vi "Main-National.vi"() -> ()   [LabVIEW 2019]
uses:
  ctl/main data-national.ctl
  ctl/position set.ctl
  ctl/act seq name.ctl
  FPGA_subVIs/low level/DIO/DIO enum.ctl
  ctl/servo act.ctl
  ctl/align type.ctl
  ctl/path name.ctl
  ctl/height.ctl
  subVI/move/position cluster.ctl
  FPGA_subVIs/low level/DIO/DIO.lvclass
  FPGA_subVIs/my FPGA lib.lvlib
panel:
  out "main-national data":T1={"board vision"=[["green", "", "", ""], ["black", "", "", ""], ["", "", "", "yellow"], ["blue", "", "", ""], ["red", "", "", ""]], "recycle room"=[], "box array"=[], "catch array"=[], "put room"="", "catch count"=0.0, "position set"={"vision board"=0.0, "catch box"=0.0, "R1 position"=0.0, "R5 position"=0.0}, "reg data"=[], "S gyro"=0.0}
  out "error out":errorcluster
  in  "error in (no error)":errorcluster
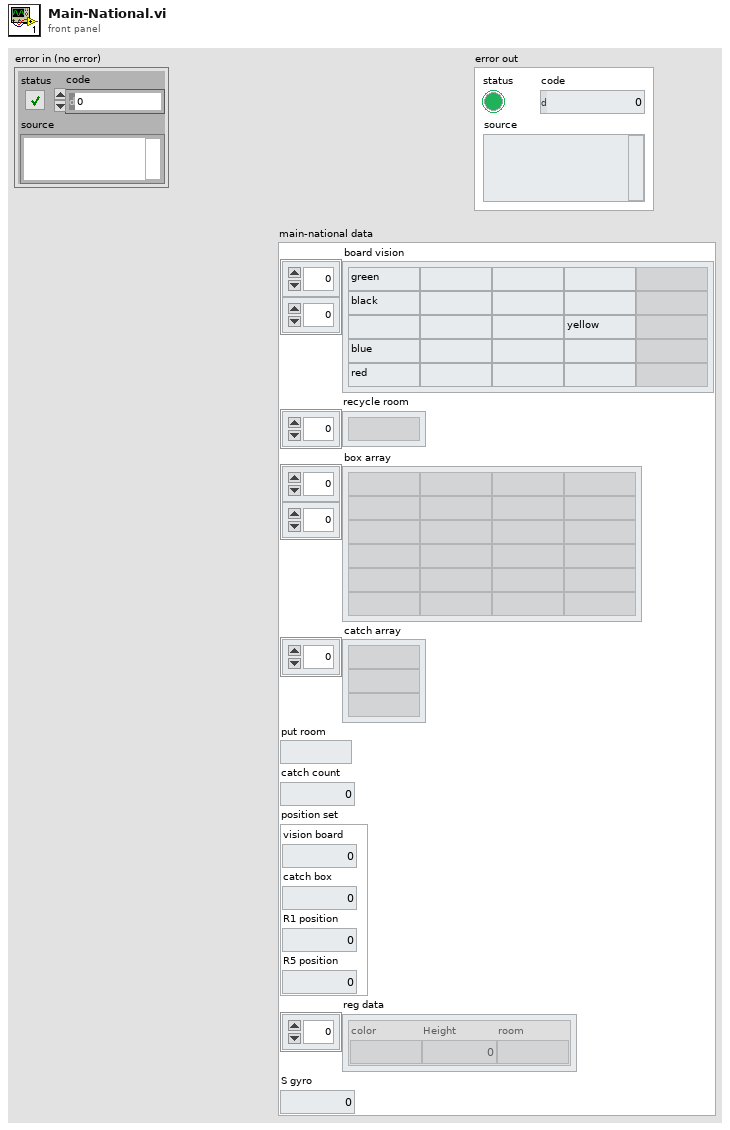
[diagram p1: front panel]
types:
  T1 = typedef "main data-national.ctl" = cluster{"board vision":string[][], "recycle room":string[], "box array":string[][], "catch array":string[], "put room":string, "catch count":dbl, "position set":T2, "reg data":cluster{"color":string, "Height":i32, "room":string}[], "S gyro":dbl}
  T2 = typedef "position set.ctl" = cluster{"vision board":dbl, "catch box":dbl, "R1 position":dbl, "R5 position":dbl}
  T3 = typedef "act seq name.ctl" = enum16{"init", "goto vision board", "go room for get recycle", "go recycle zone", "recycle go home", "goto box&room", "box act"}
  T4 = typedef "my FPGA lib.lvlib/DIO.lvclass/DIO enum.ctl" = enum16{"US.1", "US.2", "US.3", "US.4", "H.1", "H.2", "H.3", "H.4", "H.5"}
  T5 = typedef "align type.ctl" = enum16{"S zone", "box align", "box align contrast", "R1 align", "R5 align", "-> R5 center align", "-> R1 center align"}
  T6 = typedef "servo act.ctl" = enum16{"catch", "relax", "left idle", "center", "red relax", "left reg", "right reg"}
  T7 = typedef "height.ctl" = enum16{"IDLE", "recycle pre-catch", "recycle catch", "recycle zone", "vision height", "box 1", "box 2", "box 3", "box 1 pre", "box 2 pre", "box 3 pre", "reg 1", "reg 2", "reg 1 pre", "reg 2 pre", "put 1", "put 2", "put 3"}
  T8 = typedef "position cluster.ctl" = cluster{"X":dbl, "Y":dbl, "Angle":dbl}
  T9 = typedef "path name.ctl" = enum16{"S - vision board", "vision board - s out", "s out - room center", "room center - R1", "room center - R2", "room center - R3", "room center - R4", "room center - R5", "R1 - room center", "R2 - room center", "R3 - room center", "R4 - room center", "R5 - room center", "room center - S out", "S-out - recycle", "recycle - S-out", "S-out - s", "s - s-out", "board - box", "box - board", "S out - board", "R1 - R1 d", "R5d - R5", "R3.4-R3", "R3 - R3.2", "- align", "- align.5", "R2 - R2.d", "center align"}
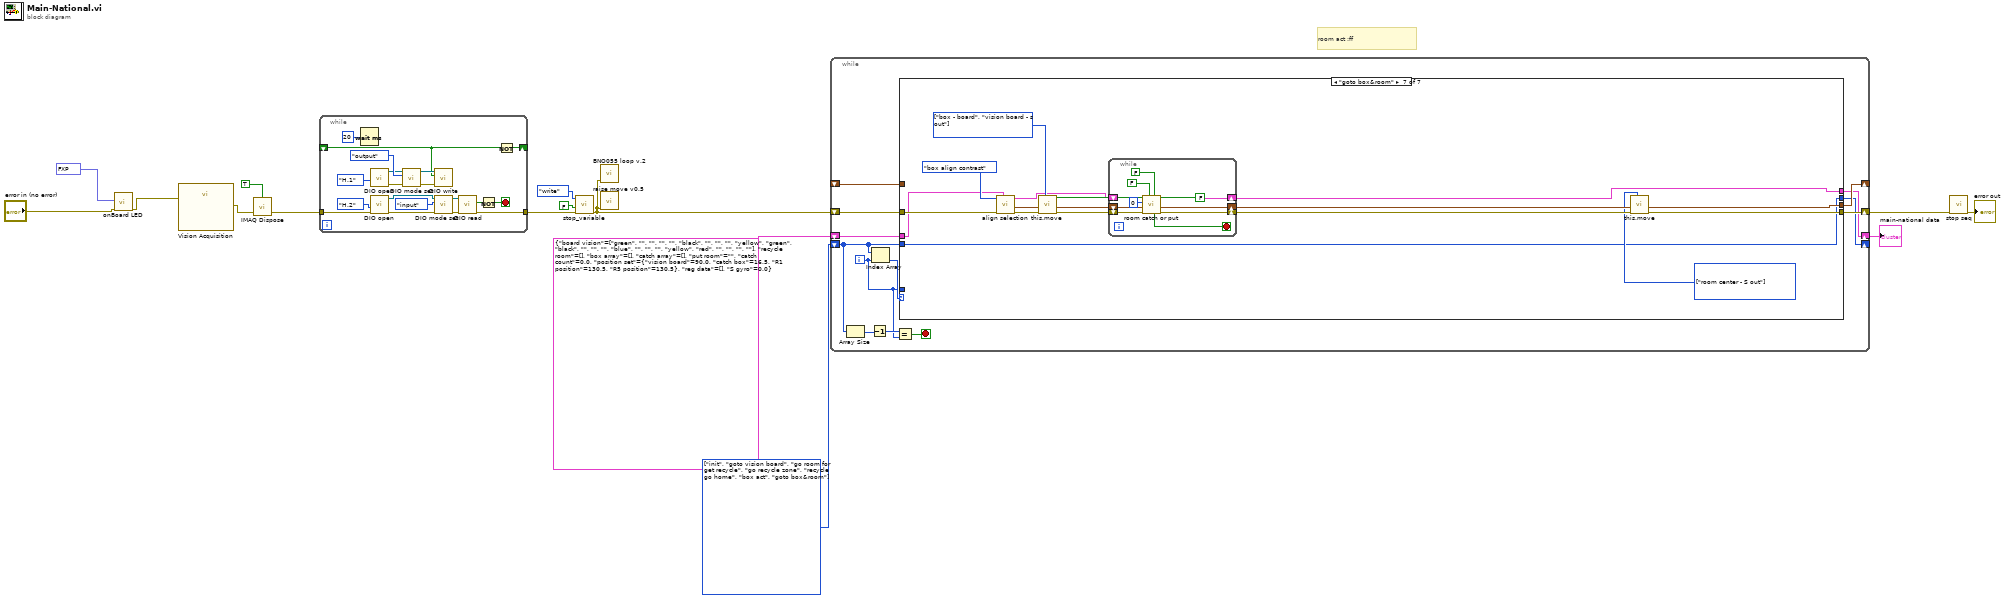
[diagram p0: block diagram]
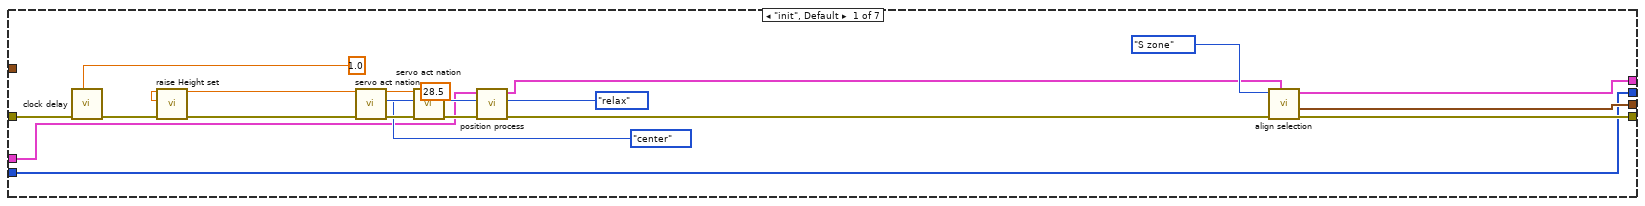
[diagram p2: hidden frame]
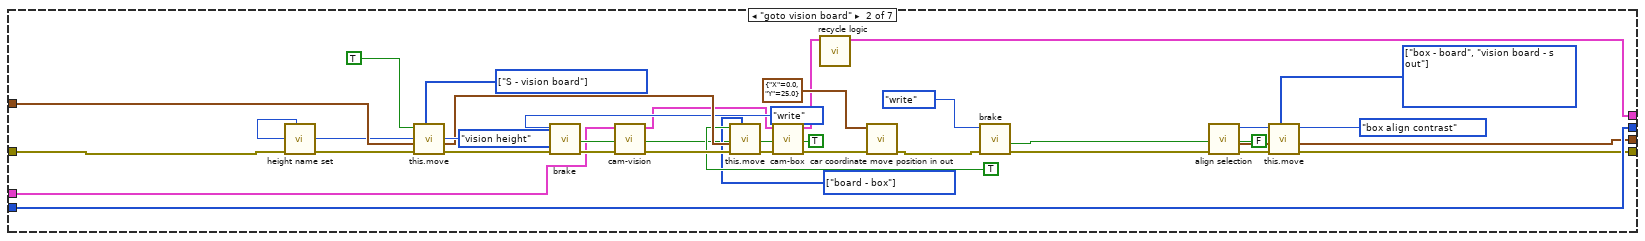
[diagram p3: hidden frame]
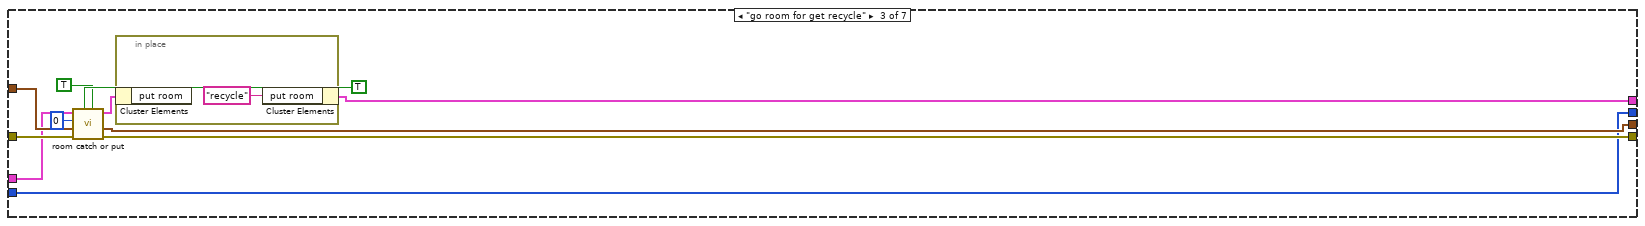
[diagram p4: hidden frame]
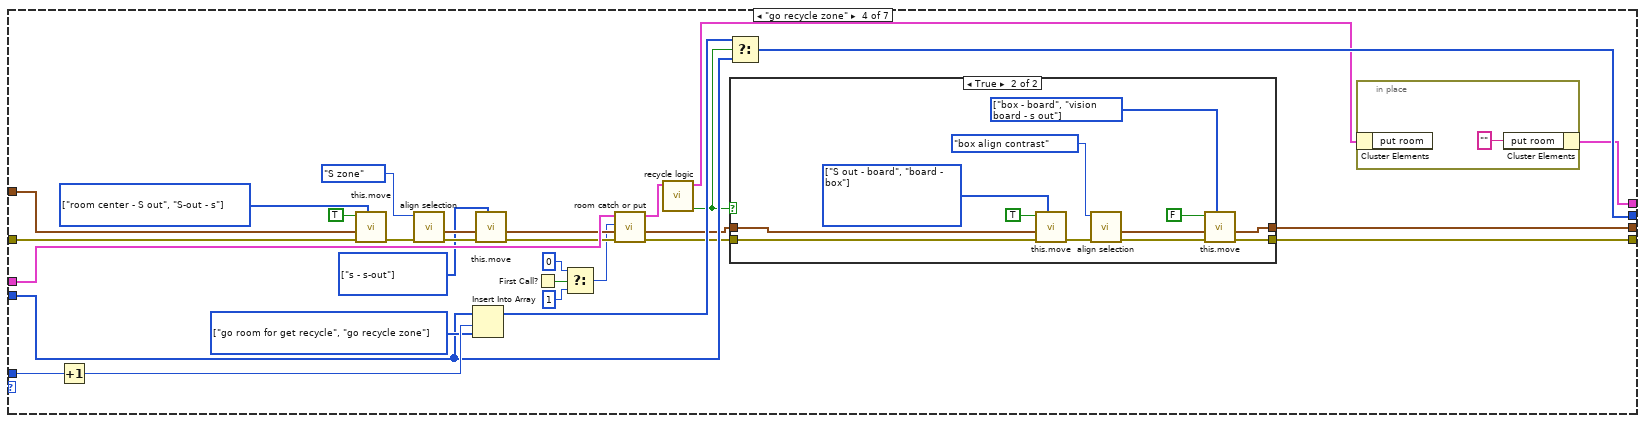
[diagram p5: hidden frame]
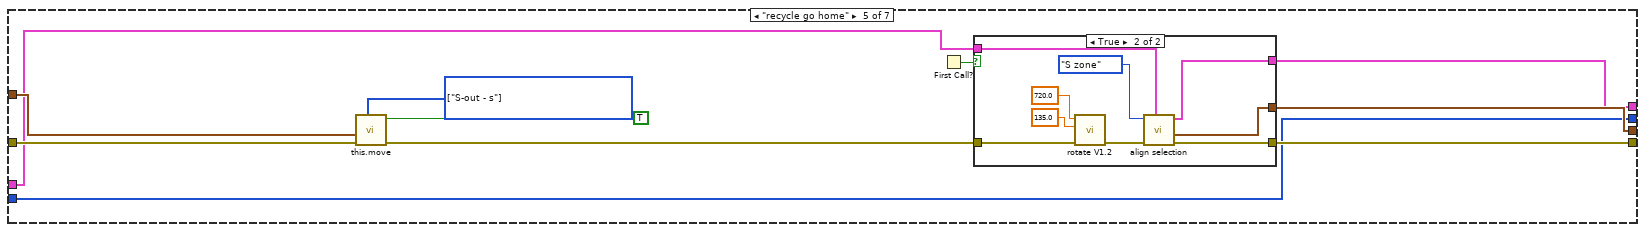
[diagram p7: hidden frame]
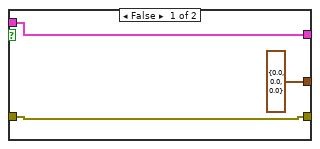
[diagram p8: hidden frame]
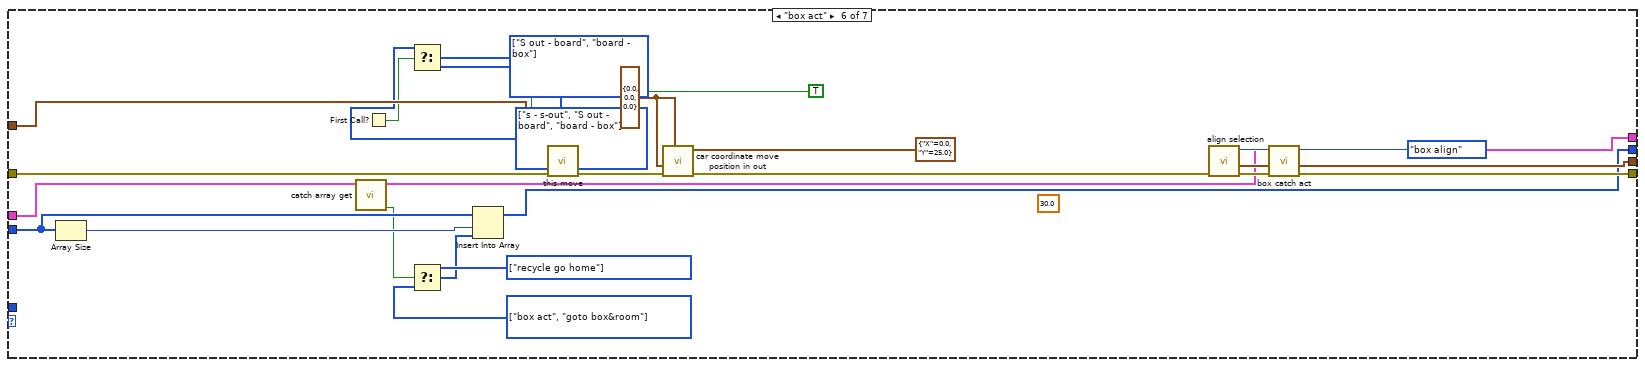
[diagram p9: hidden frame]
diagram:
  w8 = T3[] [enum."init", enum."goto vision board", enum."go room for get recycle", enum."go recycle zone", enum."recycle go home", enum."box act", enum."goto box&room"] items=["init", "goto vision board", "go room for get recycle", "go recycle zone", "recycle go home", "goto box&room", "box act"]
  # "room act :ff"
  n1 = call "onBoard LED.vi"("error in"="error in (no error)", "OnBoard.LED[3:0]"=fxp<+,4,4> 9.0) -> ("error out"=w2:errorcluster)  [unwired: 9 in]
  n2 = call "Vision Acquisition"("error in"=w2) -> ("error out"=w6:errorcluster)  [unwired: 25 in, 1 out]
  n3 = call "IMAQ Dispose"("All Images? (No)"=TRUE, "error in (no error)"=w6) -> ("error out"=w5:errorcluster)  [unwired: 4 in]
  n4 = while {
    tunnel: w5 -> [w28]
    tunnel: [w26] -> w7
    shift-right: [w17] -> _
    shift-left: _ -> [w16]
    stop <- w25 stop-if-true
    n5 = Wait (ms)(milliseconds to wait=u32 20) -> ()  [unwired: 1 out]
    n6 = call "DIO open.vi"("DIO reference"=DIO_enum."H.1") -> ("error out"=w21:errorcluster, "my FPGA lib.lvlib:DIO.lvclass"=w22:refnum<class "DIO.lvclass">)  [unwired: 9 in]
    n7 = call "DIO open.vi"("error in"=w28, "DIO reference"=DIO_enum."H.2") -> ("error out"=w33:errorcluster, "my FPGA lib.lvlib:DIO.lvclass"=w32:refnum<class "DIO.lvclass">)  [unwired: 8 in]
    n8 = call "DIO mode set.vi"("error in (no error)"=w21, "mode"=enum16{"input", "output"}."output", "DIO in"=w22) -> ("error out"=w18:errorcluster, "DIO out"=w19:refnum<class "DIO.lvclass">)  [unwired: 7 in]
    n9 = call-dynamic "DIO write.vi"("error in (no error)"=w18, "output"=w16, "DIO in"=w19) -> ()  [unwired: 7 in, 2 out]
    n10 = call "DIO mode set.vi"("error in (no error)"=w33, "mode"=enum16{"input", "output"}."input", "DIO in"=w32) -> ("error out"=w29:errorcluster, "DIO out"=w30:refnum<class "DIO.lvclass">)  [unwired: 7 in]
    n11 = call-dynamic "DIO read.vi"("error in (no error)"=w29, "DIO in"=w30) -> ("error out"=w26:errorcluster, "read"=w27:bool)  [unwired: 7 in, 1 out]
    n12 = Not(x=w27) -> (.not. x?=w25:bool)
    n13 = Not(x=w16) -> (.not. x?=w17:bool)
  }
  n14 = call "stop_variable.vi"("Error In"=w7, "Write"=FALSE, "Enum"=enum16{"read", "write"}."write") -> ("Error Out"=w12:errorcluster)  [unwired: 7 in, 1 out]
  n15 = call "BNO055 loop v.2.vi"("error in (no error)"=w12) -> ()  [unwired: 11 in]
  n16 = call "raise move v0.5.vi"("error in (no error)"=w12) -> ()  [unwired: 10 in, 1 out]
  n17 = while {
    shift-right: [w45] -> w15
    shift-left: w12 -> [w46]
    shift-right: [w44] -> _
    shift-left: _ -> [w43]
    shift-right: [w38] -> w9
    shift-left: T1 {"board vision"=[["green", "", "", "", ""], ["black", "", "", "", "yellow"], ["green", "black", "", "", ""], ["blue", "", "", "", "yellow"], ["red", "", "", "", ""]], "recycle room"=[], "box array"=[], "catch array"=[], "put room"="", "catch count"=0.0, "position set"={"vision board"=90.0, "catch box"=16.5, "R1 position"=130.5, "R5 position"=130.5}, "reg data"=[], "S gyro"=0.0} ("main-national data") -> [w39]
    shift-right: [w36] -> _
    shift-left: w8 -> [w37]
    i -> [w35]
    stop <- w40 stop-if-true
    n18 = Array Size(array=w37) -> (size(s)=w42:i32)
    n19 = Decrement(x=w42) -> (x-1=w41:i32)
    n20 = Index Array(array=w37, index=w35) -> (element=w47:T3)
    n21 = Equal?(x=w41, y=w35) -> (x = y?=w40:bool)
    n22 = case shown="\"goto box&room\"" w47 {
      tunnel: w46 -> [w64 w94 w106 w137 w164 w194 w218]
      tunnel: [w55 w70 w104 w115 w158 w199 w212] -> w44
      tunnel: [w54 w69 w105 w116 w159 w198 w213] -> w45
      tunnel: w43 -> [_ w96 w107 w136 w163 w193 _]
      tunnel: w39 -> [w50 w66 w99 w138 w155 w201 w203]
      tunnel: [w48 w67 w100 w110 w154 w189 w219] -> w38
      tunnel: w37 -> [w53 w82 w103 w121 w156 w187 w211]
      tunnel: [w53 w82 w103 w120 w156 w182 w211] -> w36
      tunnel: w35 -> [_ _ _ w125 _ _ _]
      frame "init", Default {
        n23 = call "clock delay.vi"("Delay Time (s)"=1.0, "error in (no error)"=w64) -> ("error out"=w62:errorcluster)  [unwired: 9 in]
        n24 = call "raise Height set.vi"("error in (no error)"=w62, "Height_cm"=28.5) -> ("error out"=w60:errorcluster)  [unwired: 9 in]
        n25 = call "servo act nation.vi"("error in"=w60, "servo act"=servo_act."relax") -> ("error out"=w58:errorcluster)  [unwired: 9 in]
        n26 = call "servo act nation.vi"("error in"=w58, "servo act"=servo_act."center") -> ("error out"=w52:errorcluster)  [unwired: 9 in]
        n27 = call "position process.vi"("Error In"=w52, "main-national data in"=w50) -> ("Error Out"=w51:errorcluster, "main-national data out"=w49:T1)  [unwired: 8 in]
        n28 = call "align selection.vi"("main-national data"=w49, "error in (no error)"=w51, "align type"=align_type."S zone") -> ("error out"=w54:errorcluster, "Position"=w55:T8, "main-national data out"=w48:T1)  [unwired: 6 in]
      }
      frame "goto vision board" {
        w71 = T9[] [enum."box - board", enum."vision board - s out"] items=["S - vision board", "vision board - s out", "s out - room center", "room center - R1", "room center - R2", "room center - R3", "room center - R4", "room center - R5", "R1 - room center", "R2 - room center", "R3 - room center", "R4 - room center", "R5 - room center", "room center - S out", "S-out - recycle", "recycle - S-out", "S-out - s", "s - s-out", "board - box", "box - board", "S out - board", "R1 - R1 d", "R5d - R5", "R3.4-R3", "R3 - R3.2", "- align", "- align.5", "R2 - R2.d", "center align"] ("path array")
        w87 = T9[] [enum."board - box"] items=["S - vision board", "vision board - s out", "s out - room center", "room center - R1", "room center - R2", "room center - R3", "room center - R4", "room center - R5", "R1 - room center", "R2 - room center", "R3 - room center", "R4 - room center", "R5 - room center", "room center - S out", "S-out - recycle", "recycle - S-out", "S-out - s", "s - s-out", "board - box", "box - board", "S out - board", "R1 - R1 d", "R5d - R5", "R3.4-R3", "R3 - R3.2", "- align", "- align.5", "R2 - R2.d", "center align"] ("path array")
        w95 = T9[] [enum."S - vision board"] items=["S - vision board", "vision board - s out", "s out - room center", "room center - R1", "room center - R2", "room center - R3", "room center - R4", "room center - R5", "R1 - room center", "R2 - room center", "R3 - room center", "R4 - room center", "R5 - room center", "room center - S out", "S-out - recycle", "recycle - S-out", "S-out - s", "s - s-out", "board - box", "box - board", "S out - board", "R1 - R1 d", "R5d - R5", "R3.4-R3", "R3 - R3.2", "- align", "- align.5", "R2 - R2.d", "center align"] ("path array")
        n29 = call "height name set.vi"("height name"=height."vision height", "error in (no error)"=w94) -> ("error out"=w93:errorcluster)  [unwired: 9 in]
        n30 = call "this.move.vi"("path array"=w95, "error in (no error)"=w93, "Position in"=w96, "enable"=TRUE) -> ("error out"=w81:errorcluster, "Position out"=w90:T8)  [unwired: 4 in, 2 out]
        n31 = call "brake.vi"("Error In"=w81, "write"=TRUE, "Enum"=enum16{"read", "write"}."write") -> ("Error Out"=w80:errorcluster)  [unwired: 7 in, 1 out]
        n32 = call "cam-vision.vi"("error in"=w80, "main-national data in"=w66) -> ("error out"=w89:errorcluster, "main-national data out"=w65:T1)  [unwired: 7 in, 1 out]
        n33 = call "this.move.vi"("path array"=w87, "error in (no error)"=w89, "Position in"=w90, "enable"=TRUE) -> ("error out"=w86:errorcluster)  [unwired: 4 in, 3 out]
        n34 = call "cam-box.vi"("error in"=w86, "main-national data"=w65) -> ("error out"=w84:errorcluster, "main data out"=w68:T1)  [unwired: 8 in]
        n35 = call "recycle logic.vi"("main-national data in"=w68) -> ("main-national data out"=w67:T1)  [unwired: 9 in, 1 out]
        n36 = call "car coordinate move position in out.vi"("error in (no error)"=w84, "move"=cluster{"X":dbl, "Y":dbl} {"X"=0.0, "Y"=25.0}) -> ("error out"=w77:errorcluster)  [unwired: 8 in, 1 out]
        n37 = call "brake.vi"("Error In"=w77, "write"=FALSE, "Enum"=enum16{"read", "write"}."write") -> ("Error Out"=w74:errorcluster)  [unwired: 7 in, 1 out]
        n38 = call "align selection.vi"("error in (no error)"=w74, "align type"=align_type."box align contrast") -> ("error out"=w73:errorcluster, "Position"=w72:T8)  [unwired: 7 in, 1 out]
        n39 = call "this.move.vi"("path array"=w71, "error in (no error)"=w73, "Position in"=w72) -> ("error out"=w69:errorcluster, "Position out"=w70:T8)  [unwired: 5 in, 2 out]
      }
      frame "go room for get recycle" {
        n40 = call "room catch or put.vi"("get recy?"=TRUE, "first?"=TRUE, "error in (no error)"=w106, "Position in"=w107, "ff"=0, "main-national data"=w99) -> ("error out"=w105:errorcluster, "Position out"=w104:T8, "main-national data out"=w102:T1)  [unwired: 2 in, 1 out]
        n41 = in-place {
          n42 = in-place-cluster #1(w102) -> ()  [unwired: 1 out]
          n43 = in-place-cluster #1("put room"="recycle") -> (w100:T1)
        }
      }
      frame "go recycle zone" {
        w123 = T3[] [enum."go room for get recycle", enum."go recycle zone"] items=["init", "goto vision board", "go room for get recycle", "go recycle zone", "recycle go home", "goto box&room", "box act"] ("new element/subarray")
        w129 = T9[] [enum."s - s-out"] items=["S - vision board", "vision board - s out", "s out - room center", "room center - R1", "room center - R2", "room center - R3", "room center - R4", "room center - R5", "R1 - room center", "R2 - room center", "R3 - room center", "R4 - room center", "R5 - room center", "room center - S out", "S-out - recycle", "recycle - S-out", "S-out - s", "s - s-out", "board - box", "box - board", "S out - board", "R1 - R1 d", "R5d - R5", "R3.4-R3", "R3 - R3.2", "- align", "- align.5", "R2 - R2.d", "center align"] ("path array")
        w134 = T9[] [enum."room center - S out", enum."S-out - s"] items=["S - vision board", "vision board - s out", "s out - room center", "room center - R1", "room center - R2", "room center - R3", "room center - R4", "room center - R5", "R1 - room center", "R2 - room center", "R3 - room center", "R4 - room center", "R5 - room center", "room center - S out", "S-out - recycle", "recycle - S-out", "S-out - s", "s - s-out", "board - box", "box - board", "S out - board", "R1 - R1 d", "R5d - R5", "R3.4-R3", "R3 - R3.2", "- align", "- align.5", "R2 - R2.d", "center align"] ("path array")
        n44 = Increment(x=w125) -> (x+1=w124:i32)
        n45 = call "this.move.vi"("path array"=w134, "error in (no error)"=w137, "Position in"=w136, "enable"=TRUE) -> ("error out"=w133:errorcluster)  [unwired: 4 in, 3 out]
        n46 = call "align selection.vi"("error in (no error)"=w133, "align type"=align_type."S zone") -> ("error out"=w131:errorcluster, "Position"=w130:T8)  [unwired: 7 in, 1 out]
        n47 = Insert Into Array(array=w121, index=w124, new element=w123) -> (w122:T3[])
        n48 = call "this.move.vi"("path array"=w129, "error in (no error)"=w131, "Position in"=w130) -> ("error out"=w128:errorcluster, "Position out"=w127:T8)  [unwired: 5 in, 2 out]
        n49 = First Call?() -> (First Call?: T/F=w113:bool)
        n50 = Select(t=0, s=w113, f=1) -> (s? t:f=w114:i32)
        n51 = call "room catch or put.vi"("error in (no error)"=w128, "Position in"=w127, "ff"=w114, "main-national data"=w138) -> ("error out"=w118:errorcluster, "Position out"=w117:T8, "main-national data out"=w126:T1)  [unwired: 4 in, 1 out]
        n52 = call "recycle logic.vi"("main-national data in"=w126) -> ("next?"=w119:bool, "main-national data out"=w109:T1)  [unwired: 9 in]
        n53 = Select(t=w122, s=w119, f=w121) -> (s? t:f=w120:T3[])
        n54 = case shown="True" w119 {
          tunnel: w118 -> [w141 w153]
          tunnel: w117 -> [w140 w152]
          tunnel: [w141 w144] -> w116
          tunnel: [w140 w143] -> w115
          frame False {
          }
          frame True {
            w147 = T9[] [enum."box - board", enum."vision board - s out"] items=["S - vision board", "vision board - s out", "s out - room center", "room center - R1", "room center - R2", "room center - R3", "room center - R4", "room center - R5", "R1 - room center", "R2 - room center", "R3 - room center", "R4 - room center", "R5 - room center", "room center - S out", "S-out - recycle", "recycle - S-out", "S-out - s", "s - s-out", "board - box", "box - board", "S out - board", "R1 - R1 d", "R5d - R5", "R3.4-R3", "R3 - R3.2", "- align", "- align.5", "R2 - R2.d", "center align"] ("path array")
            w151 = T9[] [enum."S out - board", enum."board - box"] items=["S - vision board", "vision board - s out", "s out - room center", "room center - R1", "room center - R2", "room center - R3", "room center - R4", "room center - R5", "R1 - room center", "R2 - room center", "R3 - room center", "R4 - room center", "R5 - room center", "room center - S out", "S-out - recycle", "recycle - S-out", "S-out - s", "s - s-out", "board - box", "box - board", "S out - board", "R1 - R1 d", "R5d - R5", "R3.4-R3", "R3 - R3.2", "- align", "- align.5", "R2 - R2.d", "center align"] ("path array")
            n55 = call "this.move.vi"("path array"=w151, "error in (no error)"=w153, "Position in"=w152, "enable"=TRUE) -> ("error out"=w148:errorcluster)  [unwired: 4 in, 3 out]
            n56 = call "align selection.vi"("error in (no error)"=w148, "align type"=align_type."box align contrast") -> ("error out"=w145:errorcluster, "Position"=w146:T8)  [unwired: 7 in, 1 out]
            n57 = call "this.move.vi"("path array"=w147, "error in (no error)"=w145, "Position in"=w146, "enable"=FALSE) -> ("error out"=w144:errorcluster, "Position out"=w143:T8)  [unwired: 4 in, 2 out]
          }
        }
        n58 = in-place {
          n59 = in-place-cluster #2(w109) -> ()  [unwired: 1 out]
          n60 = in-place-cluster #2("put room"="") -> (w110:T1)
        }
      }
      frame "recycle go home" {
        w162 = T9[] [enum."S-out - s"] items=["S - vision board", "vision board - s out", "s out - room center", "room center - R1", "room center - R2", "room center - R3", "room center - R4", "room center - R5", "R1 - room center", "R2 - room center", "R3 - room center", "R4 - room center", "R5 - room center", "room center - S out", "S-out - recycle", "recycle - S-out", "S-out - s", "s - s-out", "board - box", "box - board", "S out - board", "R1 - R1 d", "R5d - R5", "R3.4-R3", "R3 - R3.2", "- align", "- align.5", "R2 - R2.d", "center align"] ("path array")
        n61 = call "this.move.vi"("path array"=w162, "error in (no error)"=w164, "Position in"=w163, "enable"=TRUE) -> ("error out"=w160:errorcluster)  [unwired: 4 in, 3 out]
        n62 = First Call?() -> (First Call?: T/F=w157:bool)
        n63 = case shown="True" w157 {
          tunnel: w160 -> [w167 w176]
          tunnel: [w167 w171] -> w159
          tunnel: [T8 {"X"=0.0, "Y"=0.0, "Angle"=0.0} ("Position") w170] -> w158
          tunnel: w155 -> [w165 w169]
          tunnel: [w165 w168] -> w154
          frame False {
          }
          frame True {
            n64 = call "rotate V1.2.vi"("error in (no error)"=w176, "speed"=135.0, "degree"=720.0) -> ("error out"=w173:errorcluster)  [unwired: 8 in]
            n65 = call "align selection.vi"("main-national data"=w169, "error in (no error)"=w173, "align type"=align_type."S zone") -> ("error out"=w171:errorcluster, "Position"=w170:T8, "main-national data out"=w168:T1)  [unwired: 6 in]
          }
        }
      }
      frame "box act" {
        w177 = T8 {"X"=0.0, "Y"=0.0, "Angle"=0.0} ("Position in 2")
        w178 = T9[] [enum."S out - board", enum."board - box"] items=["S - vision board", "vision board - s out", "s out - room center", "room center - R1", "room center - R2", "room center - R3", "room center - R4", "room center - R5", "R1 - room center", "R2 - room center", "R3 - room center", "R4 - room center", "R5 - room center", "room center - S out", "S-out - recycle", "recycle - S-out", "S-out - s", "s - s-out", "board - box", "box - board", "S out - board", "R1 - R1 d", "R5d - R5", "R3.4-R3", "R3 - R3.2", "- align", "- align.5", "R2 - R2.d", "center align"] ("path array")
        w183 = T3[] [enum."box act", enum."goto box&room"] items=["init", "goto vision board", "go room for get recycle", "go recycle zone", "recycle go home", "goto box&room", "box act"] ("new element/subarray")
        w186 = T3[] [enum."recycle go home"] items=["init", "goto vision board", "go room for get recycle", "go recycle zone", "recycle go home", "goto box&room", "box act"] ("new element/subarray")
        w181 = T9[] [enum."s - s-out", enum."S out - board", enum."board - box"] items=["S - vision board", "vision board - s out", "s out - room center", "room center - R1", "room center - R2", "room center - R3", "room center - R4", "room center - R5", "R1 - room center", "R2 - room center", "R3 - room center", "R4 - room center", "R5 - room center", "room center - S out", "S-out - recycle", "recycle - S-out", "S-out - s", "s - s-out", "board - box", "box - board", "S out - board", "R1 - R1 d", "R5d - R5", "R3.4-R3", "R3 - R3.2", "- align", "- align.5", "R2 - R2.d", "center align"] ("path array")
        (unwired) 30.0 ("speed")
        n66 = Array Size(array=w187) -> (size(s)=w188:i32)
        n67 = call "catch array get.vi"("main-national data"=w201) -> ("finish?"=w184:bool, "main data out"=w190:T1)  [unwired: 9 in]
        n68 = First Call?() -> (First Call?: T/F=w179:bool)
        n69 = Select(t=w181, s=w179, f=w178) -> (s? t:f=w180:T9[])
        n70 = Select(t=w186, s=w184, f=w183) -> (s? t:f=w185:T3[])
        n71 = Insert Into Array(array=w187, index=w188, new element=w185) -> (w182:T3[])
        n72 = call "this.move.vi"("path array"=w180, "error in (no error)"=w194, "Position in"=w193, "enable"=TRUE) -> ("error out"=w195:errorcluster)  [unwired: 4 in, 3 out]
        n73 = call "car coordinate move position in out.vi"("Position in 2"=w177, "error in (no error)"=w195, "Position in"=w177, "move"=cluster{"X":dbl, "Y":dbl} {"X"=0.0, "Y"=25.0}) -> ("error out"=w196:errorcluster)  [unwired: 6 in, 1 out]
        n74 = call "align selection.vi"("error in (no error)"=w196, "align type"=align_type."box align") -> ("error out"=w200:errorcluster, "Position"=w191:T8)  [unwired: 7 in, 1 out]
        n75 = call "box catch act.vi"("error in (no error)"=w200, "Position"=w191, "main-national data"=w190) -> ("error out"=w198:errorcluster, "Position out"=w199:T8, "output cluster"=w189:T1)  [unwired: 6 in]
      }
      frame "goto box&room" {
        w206 = T9[] [enum."box - board", enum."vision board - s out"] items=["S - vision board", "vision board - s out", "s out - room center", "room center - R1", "room center - R2", "room center - R3", "room center - R4", "room center - R5", "R1 - room center", "R2 - room center", "R3 - room center", "R4 - room center", "R5 - room center", "room center - S out", "S-out - recycle", "recycle - S-out", "S-out - s", "s - s-out", "board - box", "box - board", "S out - board", "R1 - R1 d", "R5d - R5", "R3.4-R3", "R3 - R3.2", "- align", "- align.5", "R2 - R2.d", "center align"] ("path array")
        w214 = T9[] [enum."room center - S out"] items=["S - vision board", "vision board - s out", "s out - room center", "room center - R1", "room center - R2", "room center - R3", "room center - R4", "room center - R5", "R1 - room center", "R2 - room center", "R3 - room center", "R4 - room center", "R5 - room center", "room center - S out", "S-out - recycle", "recycle - S-out", "S-out - s", "s - s-out", "board - box", "box - board", "S out - board", "R1 - R1 d", "R5d - R5", "R3.4-R3", "R3 - R3.2", "- align", "- align.5", "R2 - R2.d", "center align"] ("path array")
        n76 = call "align selection.vi"("main-national data"=w203, "error in (no error)"=w218, "align type"=align_type."box align contrast") -> ("error out"=w209:errorcluster, "Position"=w210:T8, "main-national data out"=w204:T1)  [unwired: 6 in]
        n77 = call "this.move.vi"("path array"=w206, "error in (no error)"=w209, "Position in"=w210, "enable"=FALSE) -> ("error out"=w208:errorcluster, "Position out"=w207:T8)  [unwired: 4 in, 2 out]
        n78 = while {
          shift-right: [w228] -> w219
          shift-left: w204 -> [w229]
          shift-right: [w226] -> w216
          shift-left: w208 -> [w224]
          shift-right: [w225] -> w215
          shift-left: w207 -> [w223]
          stop <- w222 stop-if-true
          n79 = call "room catch or put.vi"("get recy?"=FALSE, "first?"=FALSE, "error in (no error)"=w224, "Position in"=w223, "ff"=0, "main-national data"=w229) -> ("error out"=w226:errorcluster, "Position out"=w225:T8, "main-national data out"=w228:T1, "finish?"=w222:bool)  [unwired: 2 in]
        }
        n80 = call "this.move.vi"("path array"=w214, "error in (no error)"=w216, "Position in"=w215) -> ("error out"=w213:errorcluster, "Position out"=w212:T8)  [unwired: 5 in, 2 out]
      }
    }
  }
  "main-national data" <- w9
  n81 = call "stop seq.vi"("error in (no error)"=w15) -> ("error out"=→"error out":errorcluster)  [unwired: 10 in]
